vi "sub_test_asap_coupling.vi"(8 "error in":errorcluster, 9 "Averaging time (ms)":u32, 10 "I2C interface":T1, 11 "Light enables":bool[](array[boolean])) -> (0 "error out":errorcluster, 3 "Demodulated signals":sgl[][](array[numeric]))   [LabVIEW 2013]
uses:
  micron/labview/manipulator/squiggle/Host/i2c_interface.ctl
  micron/labview/manipulator/squiggle/Host/fpga_reference.ctl
panel:
  # "Light"
  # "Channel"
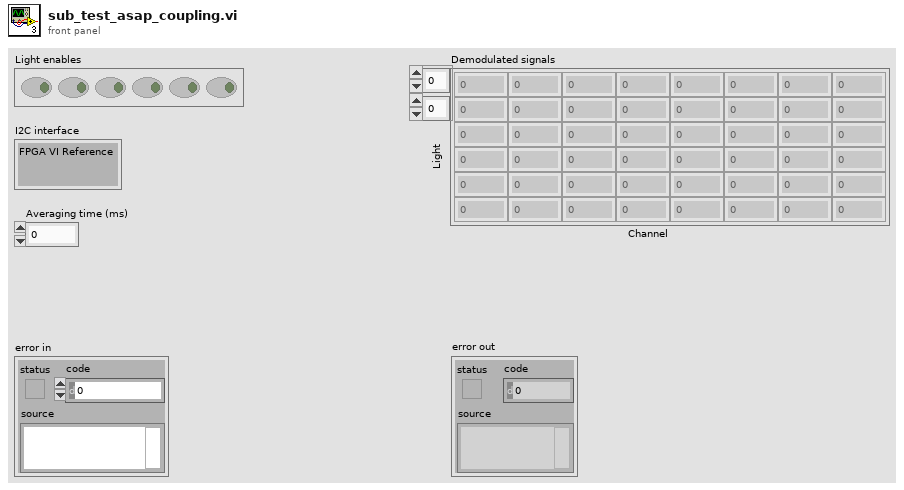
[diagram p1: front panel]
types:
  T1 = typedef "i2c_interface.ctl" = cluster{"FPGA VI Reference":T2}
  T2 = typedef "fpga_reference.ctl" = refnum<k20>
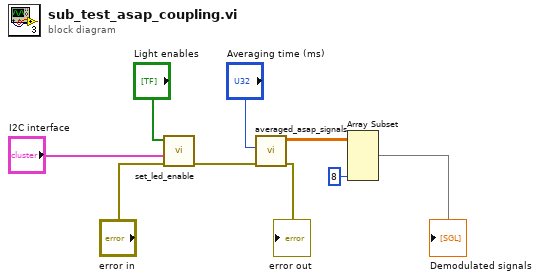
[diagram p0: block diagram]
diagram:
  n1 = call "set_led_enable.vi"("error in"="error in", "I2C interface"="I2C interface", "LED enables"="Light enables") -> ("error out"=w3:errorcluster)  [unwired: 8 in]
  n2 = call "averaged_asap_signals.vi"("error in"=w3, "Averaging time (ms)"="Averaging time (ms)") -> ("error out"=→"error out":errorcluster, "Demodulated averaged"=w6:sgl[][])  [unwired: 6 in, 2 out]
  n3 = Array Subset(array=w6, length (col)=8 ("length")) -> (→"Demodulated signals":sgl[][])  [unwired: 3 in]
